vi "Stability.vi"() -> (0 "Done!":bool)   [LabVIEW 2013]
doc: "Performs stability measurements according to ATLAS ITk Quality Control Specifications."
uses:
  InstrControl/Switching/Switching.lvclass
  InstrControl/SupplyControl/SupplyControl.lvclass
  InstrControl/MultimeterControl/MultimeterControl.lvclass
  general_VIs/globals/QC_MeasurementSetup.vi
  general_VIs/globals/QC_RunInformation.vi
  InstrControl/InstrumentSetup.vi
  InstrControl/ArduinoControl/ArduinoControl.lvclass
  InstrControl/InstrControl.lvclass
  <vilib>/Analysis/NI_AALBase.lvlib
panel:
  out "No. of sensors":i32
  out "Current":dbl[](array[numeric]) caption="Current [nA]"
  out "Tgraph":cluster{u32[], dbl[]}[](graph)
  out "Igraph":cluster{u32[], dbl[]}[](graph)
  out "Tab Control 2":enum32{"Stability Setup", "Stability Scan"}(tab)
  in  "Use DUT switch?":bool=TRUE
  in  "Add Button":bool
  in  "New Button":bool
  out "DB Serial Nos.":string[](array[string])
  out "Channel Nos.":string[](array[string])
  in  "User:":string(combo)="Christoph"
  in  "Quit":bool
  in  "Continue":bool
  in  "enable T\ncorrection":bool
  in  "Base\nTemperature":dbl=20.0 format="%.1f"
  out "scan interval [s]":i32=10
  out "Test Duration":u32 format="%<%H:%M:%S>t"
  out "Voltage [V]":dbl format="%.1f"
  out "Temp.":dbl[](array[numeric]) caption="Temp. [°C]" format="%#.2f"
  out "RH":dbl[](array[numeric]) caption="RH [%]" format="%#.2f"
  in  "Scales":T1(ring)
  in  "Iscale":enum16{"nanoAmps", "microAmps", "milliAmps"}(ring)
  out "positive ramp?":bool
  out "Tab Control":enum32{"Stability Setup", "Stability Scan"}(tab)
  in  "Temperature":enum16{"Read Arduino", "Enter manually"}(ring)
  in  "Bias Supply":string(combo)="Keithley 2410"
  in  "Hardware Configurations":bool
  in  "DMM":string(combo)="Keithley 2000"
  in  "Set current limit?":bool
  in  "Current Limit [µA]":dbl=1000.0 min=0.0001 format="%.3f"
  in  "Test Duration IN":u32 caption="Test Duration" format="%<%H:%M:%S>t"
  in  "Measurement Configurations":bool
  in  "Voltage [V] IN":dbl caption="Voltage [V]"
  in  "scan interval [s] IN":i32=10 caption="scan interval [s]"
  in  "abort":bool
  out "Current Volts:":dbl format="%.2f"
  in  "quit (no save)":bool
  in  "Quit & Save":bool
  out "Bias On/Off:":bool
  out "STATUS 1":string
  out "Initiated:":string
  out "end of run":u32 format="%<%X\n%d/%m>T"
  out "runtime":u32 format="%<%H:%M:%S>t"
  out "Last reading at:":string
  # "University of\nCambridge"
  # "Strip Sensor QC: Current Stability"
  # "Vertical Scale:"
  # "DUT Description"
  # "Stability Scan parameters:"
  # "Temperature correction:"
  # "Measurement Configuration"
  # "Hardware"
  # "Current status:"
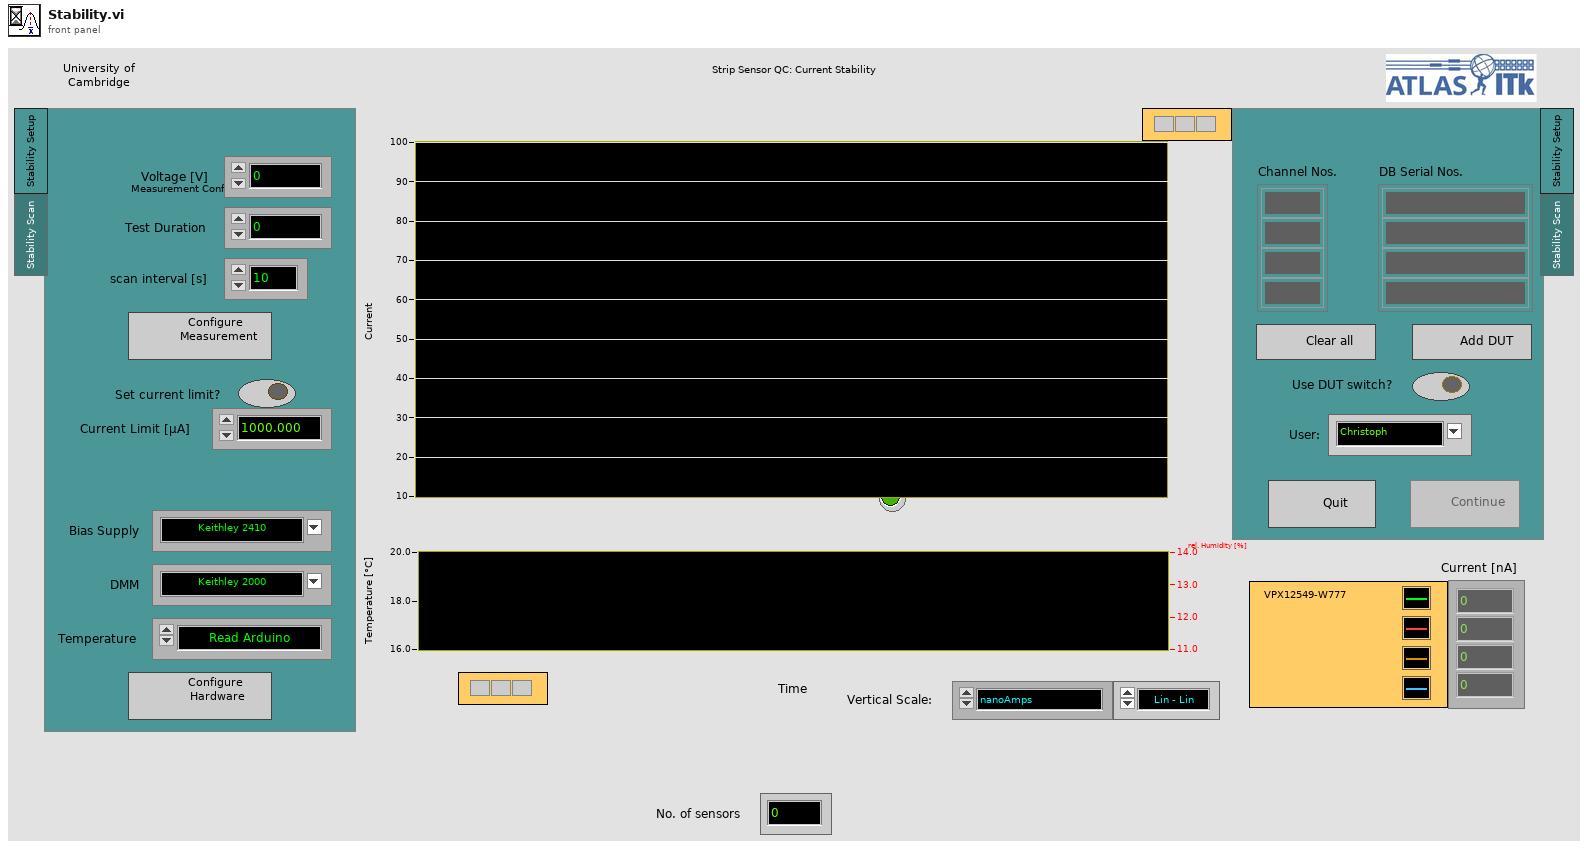
[diagram p1: front panel]
types:
  T1 = enum16{"Lin - Lin", "Log - Lin", "Lin - Log", "Log - log"}
  T2 = enum16{"Supply", "LCR", "Multimeter", "Switching"}
  T3 = enum32{"IV", "CV", "Stability", "Striptest", "Cis", "Ris", "PTP"}
  T4 = cluster{"Institute":string, "Manufacturers":string[], "Devices":string[], "Serialnumbers Lookup DB":string, "Data directory":string, "Backup & screenshot directory":string, "List of known users":string[], "Measurement switch not used":bool, "Measurement Switch":string, "DUT Switch":string, "Rseries IV [MOhm]":string, "Rshunt IV [MOhm]":string, "Rseries CV [MOhm]":string, "DC blocking Cap [µF]":string, "Rseries LCR [MOhm]":string, "Rseries stability [MOhm]":string, "Rshunt stability [MOhm]":string, "Rseries striptest bias [MOhm]":string, "Rseries strip pinhole [MOhm]":string}
  T5 = cluster{"Sensor Serial No.:":string, "Wafer:":string, "Batch:":string, "Manufacturer:":string, "Device Category:":string, "Database Serial No.:":string, "Date Initiated:":string, "Time Initiated:":string, "Test":string, "Probeplan used:":string, "End of Run comment:":string, "User:":string, "Vbias SMU":string, "LCR":string, "Test SMU":string, "Test DMM":string}
  T6 = cluster{"Supply":refnum<class "SupplyControl.lvclass">, "DMM":refnum<class "MultimeterControl.lvclass">, "DUT switch":refnum<class "Switching.lvclass">, "Arduino":refnum<class "ArduinoControl.lvclass">, "Measurement switch":refnum<class "Switching.lvclass">, "Voltage [V]":dbl, "Measurement Interval [s]":i32, "Test Duration":u32, "Ramp up steps [V]":dbl, "Ramp up Interval [s]":u32, "Ramp down steps [V]":dbl, "Ramp down Interval [s]":i32, "Set Current Limit?":bool, "Current Limit [µA]":dbl, "Temperature Readout":enum16{"Read Arduino", "Enter manually"}, "Supply Name":string, "DMM Name":string, "Maximum current fluctuation [%]":dbl, "Measurement switch used?":bool, "DUT switch used?":bool}
  T7 = enum16{"Reset", "Read Array", "Read Element", "Write Element", "Write Array", "Add Element", "Add Array"}
  T8 = cluster{"VISA address":refnum<visa-resource-name>, "T sensor":enum16{"SHT", "DS"}, "Arduino":refnum<class "ArduinoControl.lvclass">}
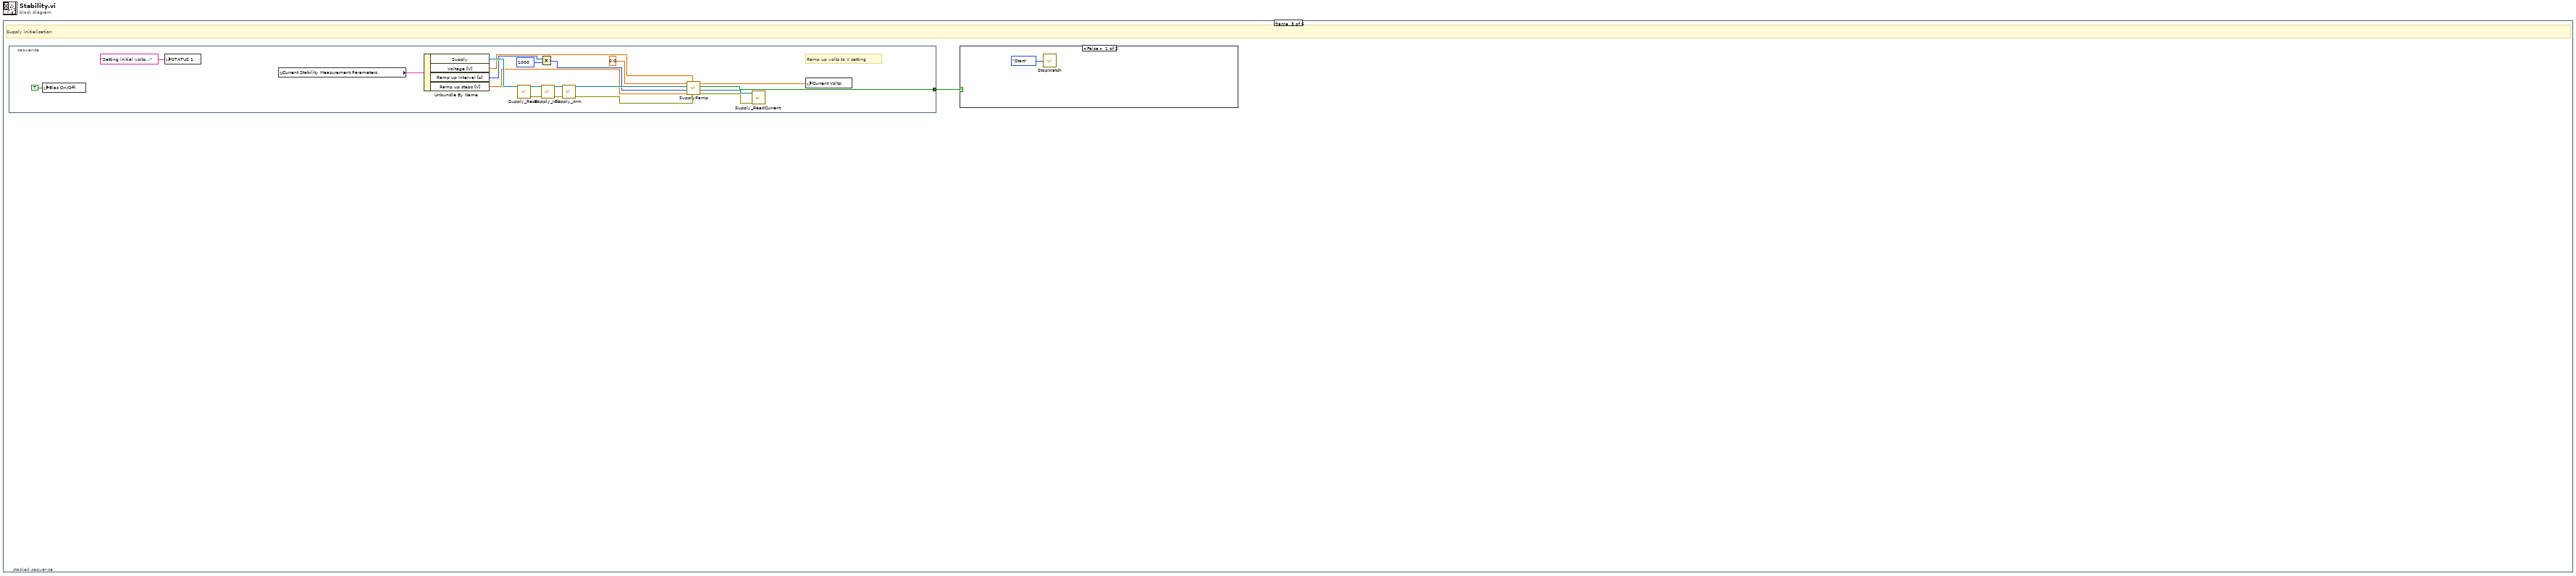
[diagram p0: block diagram]
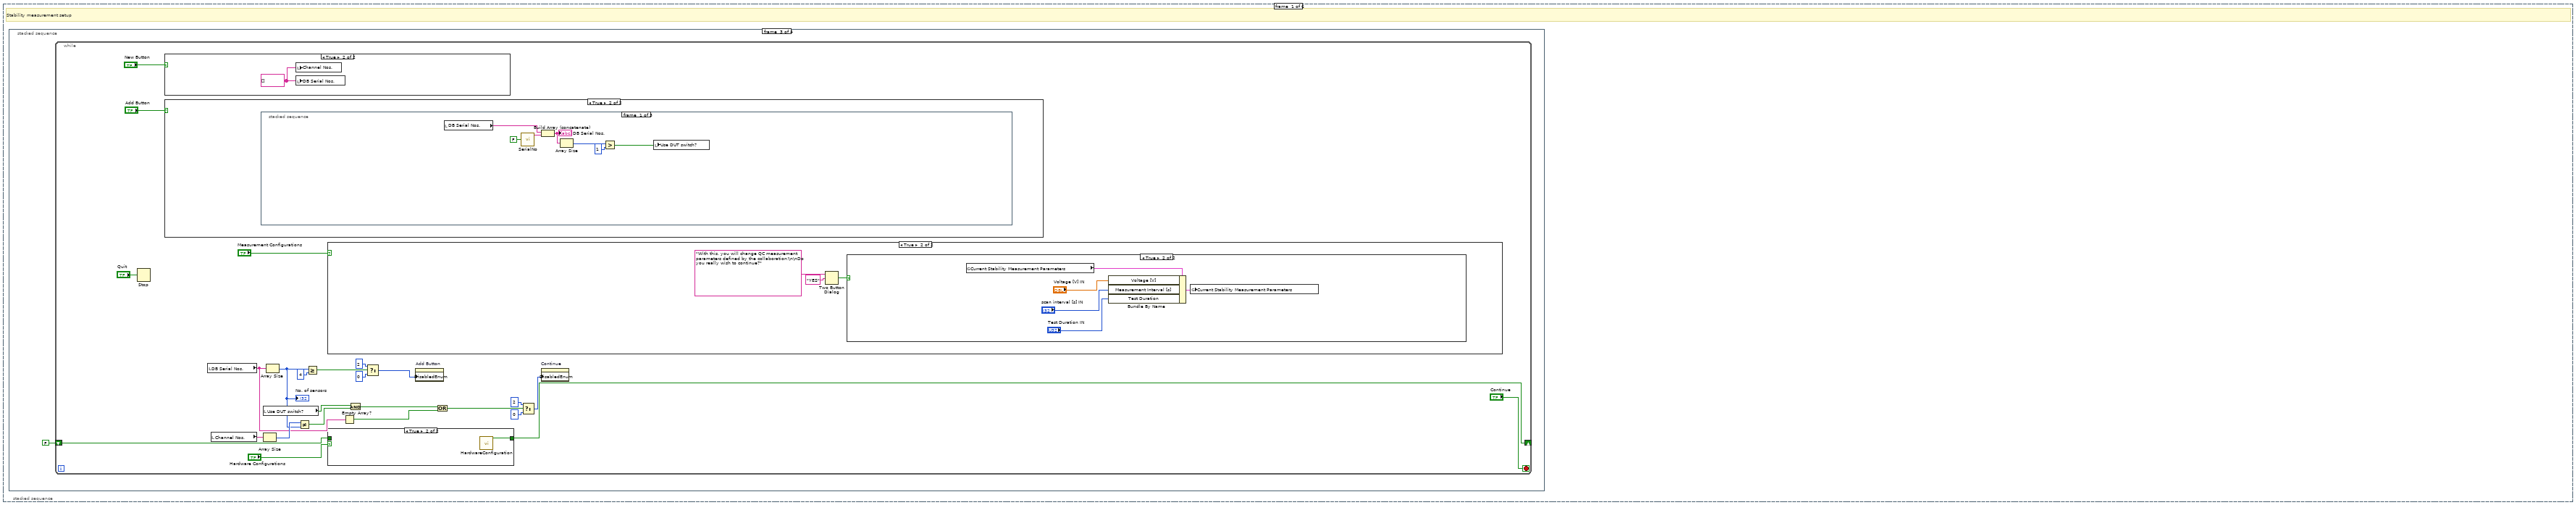
[diagram p2: hidden frame]
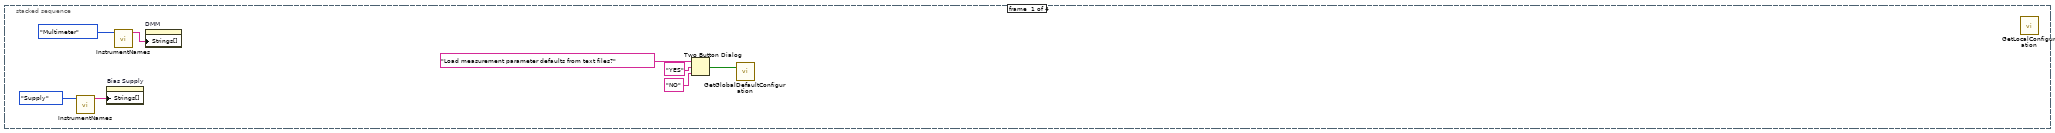
[diagram p3: hidden frame]
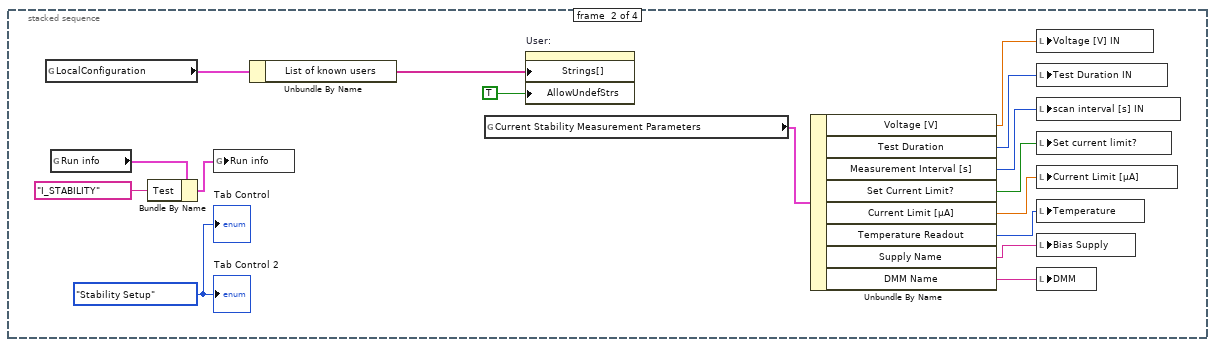
[diagram p4: hidden frame]
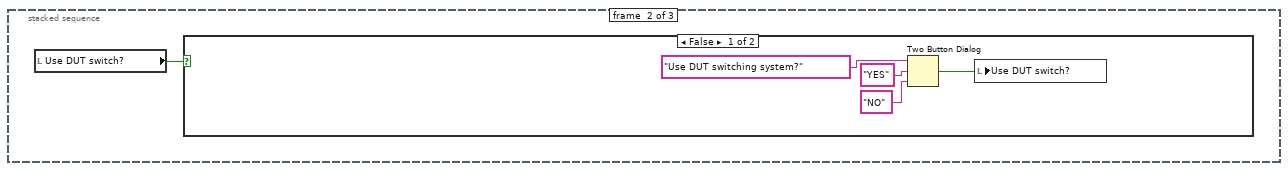
[diagram p7: hidden frame]
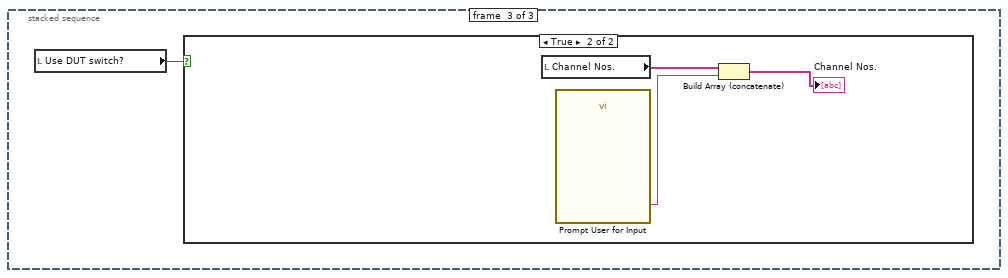
[diagram p9: hidden frame]
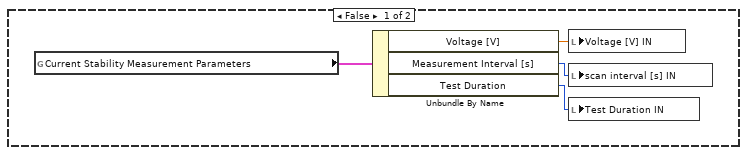
[diagram p12: hidden frame]
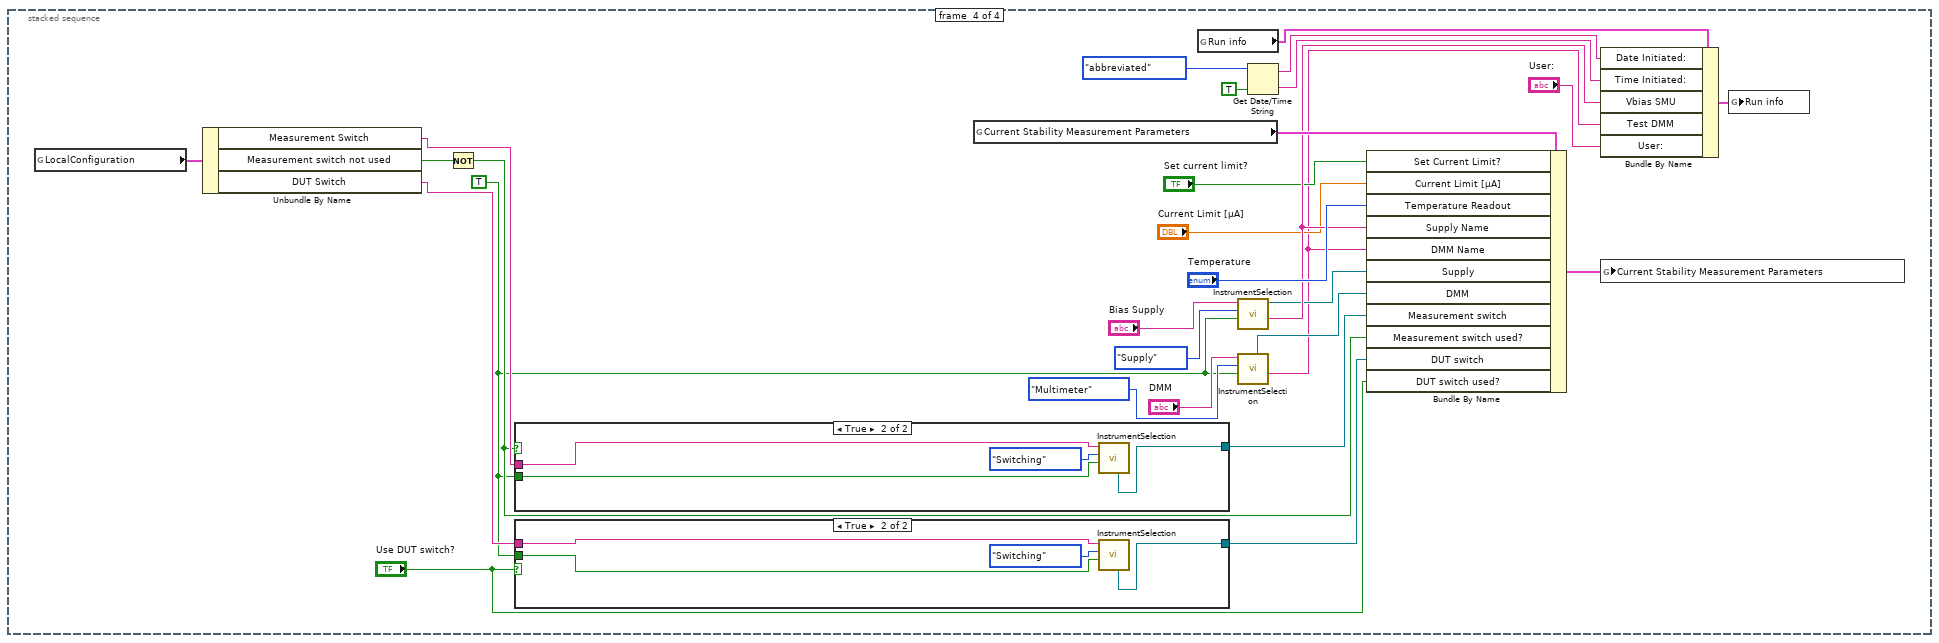
[diagram p14: hidden frame]
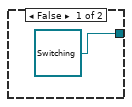
[diagram p15: hidden frame]
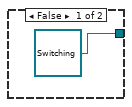
[diagram p16: hidden frame]
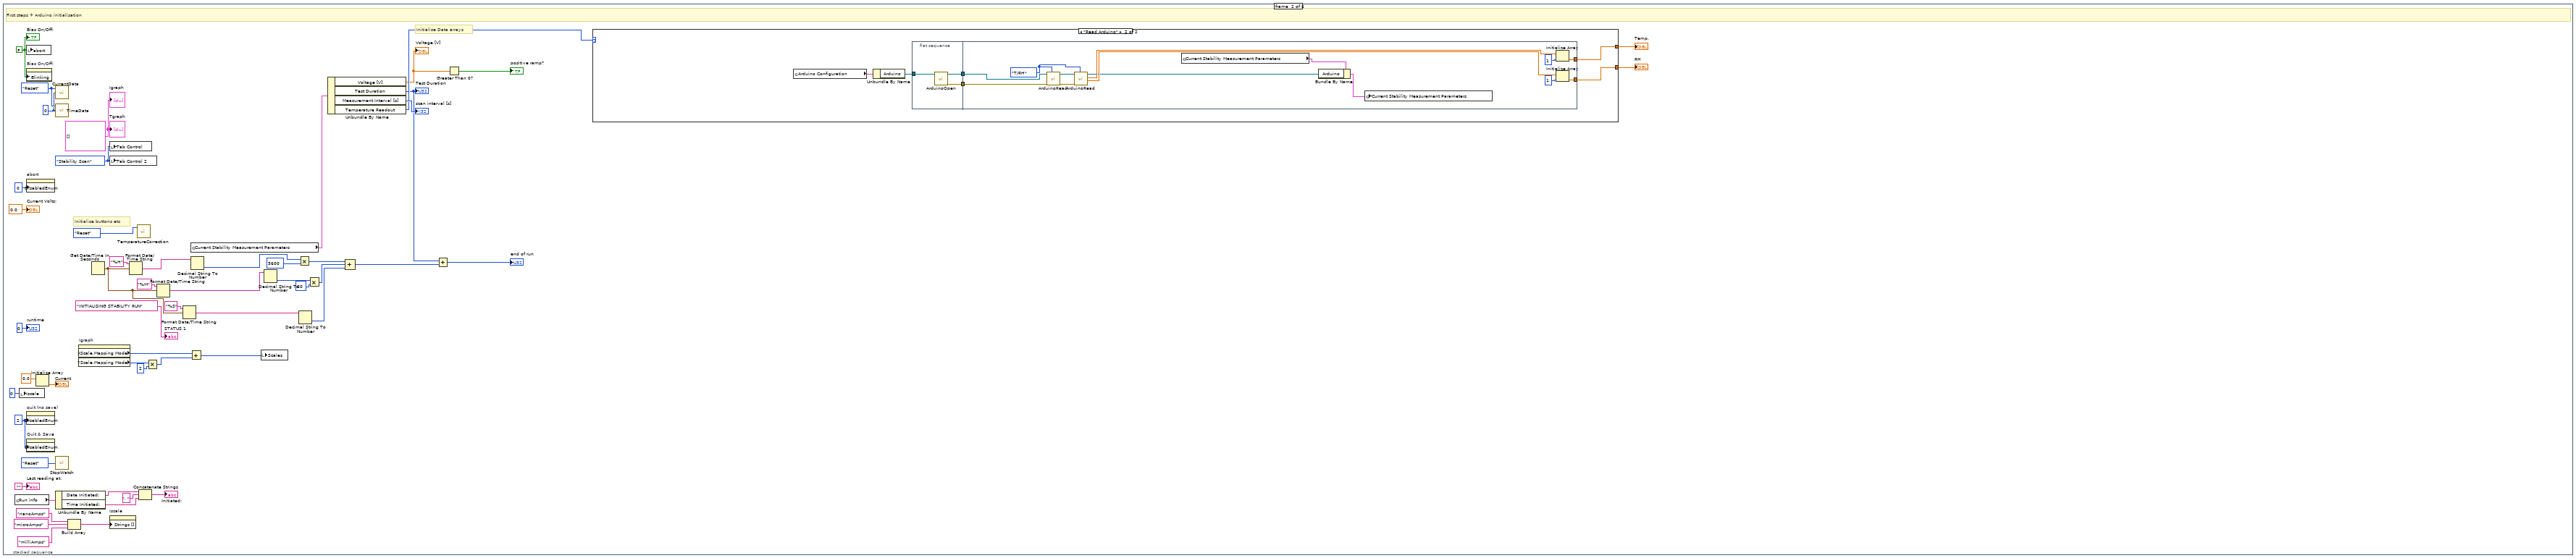
[diagram p17: hidden frame]
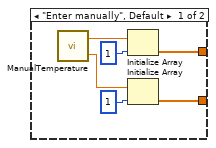
[diagram p18: hidden frame]
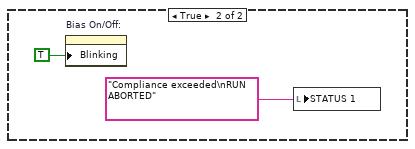
[diagram p19: hidden frame]
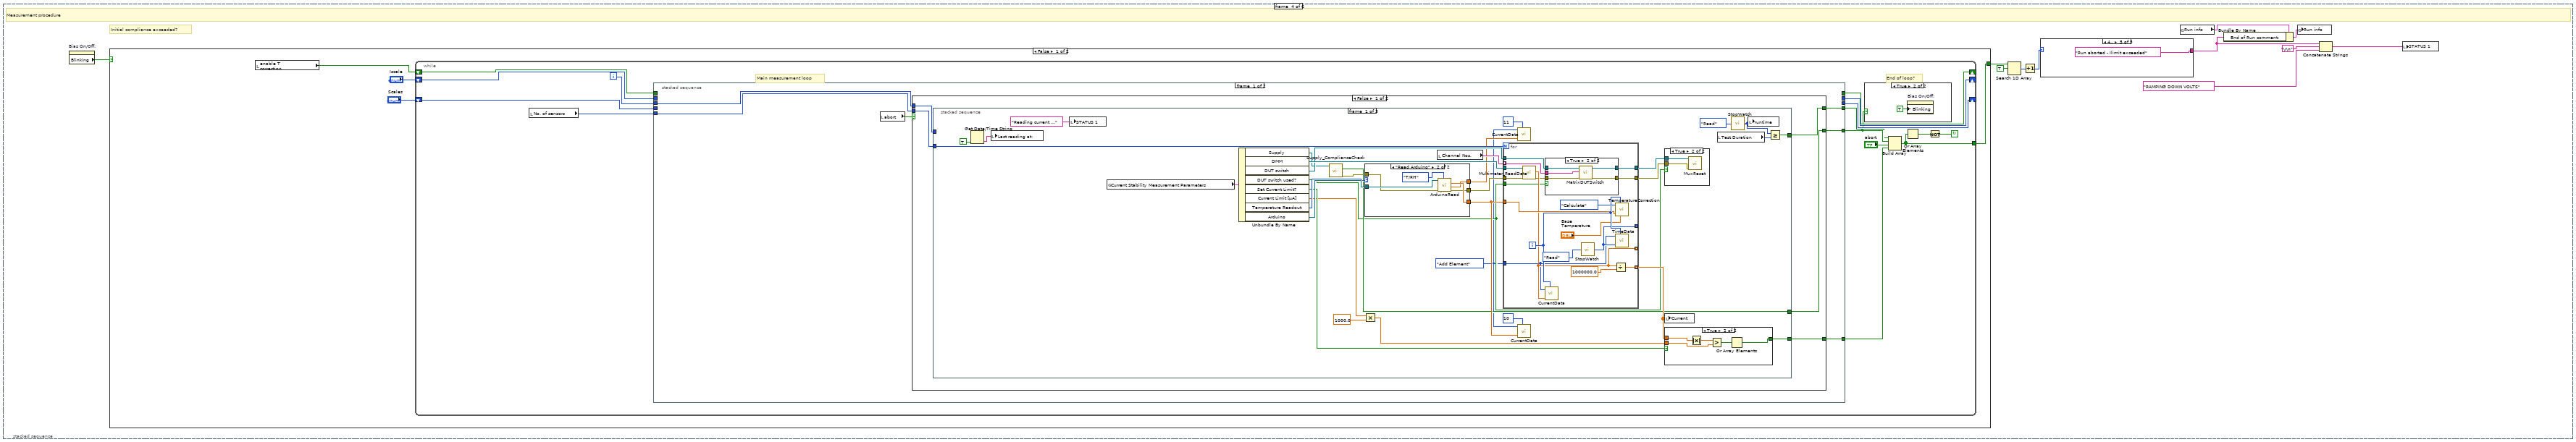
[diagram p20: hidden frame]
diagram:
  n1 = stacked-sequence {
    frame #0 {
      # "Stability measurement setup"
      n2 = stacked-sequence {
        frame #0 {
          n3 = call "InstrumentNames.vi"("Instrument type"=T2."Supply") -> ("Instrument names"=w7:string[])  [unwired: 9 in, 1 out]
          n4 = property on="Bias Supply" class="CmbBox"("Strings[]"=w7) -> ()  [unwired: 2 in, 2 out]
          n5 = call "InstrumentNames.vi"("Instrument type"=T2."Multimeter") -> ("Instrument names"=w2:string[])  [unwired: 9 in, 1 out]
          n6 = property on="DMM" class="CmbBox"("Strings[]"=w2) -> ()  [unwired: 2 in, 2 out]
          n7 = Two Button Dialog(message="Load measurement parameter defaults from text files?", 1:"NO", 2:"YES") -> (T button?=w6:bool)
          n8 = call "GetGlobalDefaultConfiguration.vi"("Read defaults?"=w6) -> ()  [unwired: 3 in]
          n9 = call "GetLocalConfiguration.vi"() -> ()  [unwired: 3 in, 1 out]
        }
        frame #1 {
          w13 = enum32{"Stability Setup", "Stability Scan"}."Stability Setup" ("Tab Control")
          n10 = global read "QC_RunInformation.vi" "LocalConfiguration"() -> (w10:T4)
          n11 = global read "QC_RunInformation.vi" "Run info"() -> (w19:T5)
          n12 = Bundle By Name(cluster=w19, "Test"="I_STABILITY") -> (w18:T5)
          n13 = global write "QC_RunInformation.vi" "Run info"(w18) -> ()
          n14 = Unbundle By Name(w10) -> ("List of known users"=w11:string[])
          n15 = global read "QC_MeasurementSetup.vi" "Current Stability Measurement Parameters"() -> (w22:T6)
          n16 = property on="User:" class="CmbBox"("Strings[]"=w11, "AllowUndefStrs"=TRUE) -> ()  [unwired: 2 in, 2 out]
          n17 = Unbundle By Name(w22) -> ("Voltage [V]"=w16:dbl, "Test Duration"=w15:u32, "Measurement Interval [s]"=w17:i32, "Set Current Limit?"=w21:bool, "Current Limit [µA]"=w20:dbl, "Temperature Readout"=w24:enum16{"Read Arduino", "Enter manually"}, "Supply Name"=w23:string, "DMM Name"=w9:string)
          n18 = local write "Voltage [V] IN"(w16) -> ()
          n19 = local write "Test Duration IN"(w15) -> ()
          n20 = local write "scan interval [s] IN"(w17) -> ()
          n21 = local write "Set current limit?"(w21) -> ()
          n22 = local write "Current Limit [µA]"(w20) -> ()
          n23 = local write "Temperature"(w24) -> ()
          n24 = local write "Bias Supply"(w23) -> ()
          n25 = local write "DMM"(w9) -> ()
          "Tab Control" <- w13
          "Tab Control 2" <- w13
        }
        frame #2 {
          n26 = while {
            shift-right: [w47] -> _
            shift-left: FALSE -> [w46]
            stop <- "Continue" stop-if-true
            n27 = Stop(stop? (T)="Quit") -> ()
            n28 = case shown="True" "New Button" {
              frame False {
              }
              frame True {
                w51 = string[] [] ("Channel Nos.")
                n29 = local write "Channel Nos."(w51) -> ()
                n30 = local write "DB Serial Nos."(w51) -> ()
              }
            }
            n31 = case shown="True" "Add Button" {
              frame False {
              }
              frame True {
                n32 = stacked-sequence {
                  frame #0 {
                    n33 = local read "DB Serial Nos."() -> (w57:string[])
                    n34 = call "SerialNo.vi"("Run uninterrupted?"=FALSE) -> ("DB serial number OUT"=w56:string)  [unwired: 7 in, 1 out]
                    n35 = Build Array (concatenate)(w57, w56) -> (w53:string[])
                    "DB Serial Nos." <- w53
                    n36 = Array Size(array=w53) -> (size(s)=w55:i32)
                    n37 = Greater?(x=w55, y=1) -> (0:w52:bool)
                    n38 = local write "Use DUT switch?"(w52) -> ()
                  }
                  frame #1 {
                    n39 = local read "Use DUT switch?"() -> (w59:bool)
                    n40 = case shown="False" w59 {
                      frame False {
                        n41 = Two Button Dialog(message="Use DUT switching system?", 1:"NO", 2:"YES") -> (T button?=w60:bool)
                        n42 = local write "Use DUT switch?"(w60) -> ()
                      }
                      frame True {
                      }
                    }
                  }
                  frame #2 {
                    n43 = local read "Use DUT switch?"() -> (w64:bool)
                    n44 = case shown="True" w64 {
                      frame False {
                      }
                      frame True {
                        n45 = local read "Channel Nos."() -> (w66:string[])
                        n46 = call "Prompt User for Input"() -> ("channel no."=w67:string)  [unwired: 17 in, 2 out]
                        n47 = Build Array (concatenate)(w66, w67) -> (→"Channel Nos.":string[])
                      }
                    }
                  }
                }
              }
            }
            n48 = local read "DB Serial Nos."() -> (w38:string[])
            n49 = local read "Channel Nos."() -> (w39:string[])
            n50 = local read "Use DUT switch?"() -> (w30:bool)
            n51 = Array Size(array=w39) -> (size(s)=w40:i32)
            n52 = Array Size(array=w38) -> (size(s)=w36:i32)
            "No. of sensors" <- w36
            n53 = Not Equal?(x=w40, y=w36) -> (x != y?=w31:bool)
            n54 = Greater Or Equal?(x=w36, y=4) -> (x >= y?=w32:bool)
            n55 = case shown="True" "Measurement Configurations" {
              frame False {
              }
              frame True {
                n56 = Two Button Dialog(message="With this, you will change QC measurement parameters defined by the collaboration!\n\nDo you really wish to continue?", 2:"YES") -> (T button?=w68:bool)  [unwired: 1 in]
                n57 = case shown="True" w68 {
                  frame False {
                    n58 = global read "QC_MeasurementSetup.vi" "Current Stability Measurement Parameters"() -> (w74:T6)
                    n59 = Unbundle By Name(w74) -> ("Voltage [V]"=w73:dbl, "Measurement Interval [s]"=w72:i32, "Test Duration"=w71:u32)
                    n60 = local write "Voltage [V] IN"(w73) -> ()
                    n61 = local write "scan interval [s] IN"(w72) -> ()
                    n62 = local write "Test Duration IN"(w71) -> ()
                  }
                  frame True {
                    n63 = global read "QC_MeasurementSetup.vi" "Current Stability Measurement Parameters"() -> (w79:T6)
                    n64 = Bundle By Name(cluster=w79, "Voltage [V]"="Voltage [V] IN", "Measurement Interval [s]"="scan interval [s] IN", "Test Duration"="Test Duration IN") -> (w78:T6)
                    n65 = global write "QC_MeasurementSetup.vi" "Current Stability Measurement Parameters"(w78) -> ()
                  }
                }
              }
            }
            n66 = case shown="True" "Hardware Configurations" {
              tunnel: [w80 w81] -> w47
              tunnel: w46 -> [w80 _]
              frame False {
              }
              frame True {
                n67 = call "HardwareConfiguration.vi"() -> ("configured?"=w81:bool)  [unwired: 11 in]
              }
            }
            n68 = Empty Array?(array=w38) -> (empty?=w29:bool)
            n69 = And(x=w30, y=w31) -> (x .and. y?=w28:bool)
            n70 = Select(t=2, s=w32, f=0) -> (s? t:f=w33:i32)
            n71 = property on="Add Button" class="Bool"("DisabledEnum"=w33) -> ()  [unwired: 2 in, 2 out]
            n72 = Or(x=w28, y=w29) -> (x .or. y?=w27:bool)
            n73 = Select(t=2, s=w27, f=0) -> (s? t:f=w43:i32)
            n74 = property on="Continue" class="Bool"("DisabledEnum"=w43) -> ()  [unwired: 2 in, 2 out]
          }
        }
        frame #3 {
          w82 = TRUE
          n75 = global read "QC_RunInformation.vi" "LocalConfiguration"() -> (w95:T4)
          n76 = Unbundle By Name(w95) -> ("Measurement Switch"=w93:string, "Measurement switch not used"=w94:bool, "DUT Switch"=w89:string)
          n77 = Not(x=w94) -> (.not. x?=w92:bool)
          n78 = case shown="True" w92 {
            tunnel: [refnum<class "Switching.lvclass"> refnum ("Switching") w119] -> w99
            tunnel: w82 -> [_ w118]
            tunnel: w93 -> [_ w117]
            frame False {
            }
            frame True {
              n79 = call "InstrumentSelection.vi"("Verify GPIB address"=w118, "Instrument type"=T2."Switching", "Instrument name IN"=w117) -> ("Switching"=w119:refnum<class "Switching.lvclass">)  [unwired: 3 in, 5 out]
            }
          }
          n80 = case shown="True" "Use DUT switch?" {
            tunnel: w89 -> [_ w114]
            tunnel: w82 -> [_ w113]
            tunnel: [refnum<class "Switching.lvclass"> refnum ("Switching") w112] -> w86
            frame False {
            }
            frame True {
              n81 = call "InstrumentSelection.vi"("Verify GPIB address"=w113, "Instrument type"=T2."Switching", "Instrument name IN"=w114) -> ("Switching"=w112:refnum<class "Switching.lvclass">)  [unwired: 3 in, 5 out]
            }
          }
          n82 = global read "QC_MeasurementSetup.vi" "Current Stability Measurement Parameters"() -> (w109:T6)
          n83 = global read "QC_RunInformation.vi" "Run info"() -> (w96:T5)
          n84 = call "InstrumentSelection.vi"("Verify GPIB address"=w82, "Instrument type"=T2."Supply", "Instrument name IN"="Bias Supply") -> ("Instrument name OUT"=w101:string, "Supply"=w100:refnum<class "SupplyControl.lvclass">)  [unwired: 3 in, 4 out]
          n85 = call "InstrumentSelection.vi"("Verify GPIB address"=w82, "Instrument type"=T2."Multimeter", "Instrument name IN"="DMM") -> ("Instrument name OUT"=w84:string, "Multimeter"=w87:refnum<class "MultimeterControl.lvclass">)  [unwired: 3 in, 4 out]
          n86 = Get Date/Time String(date format (0)=enum16{"short", "long", "abbreviated"}."abbreviated", want seconds? (F)=TRUE) -> (date string=w98:string, time string=w97:string)  [unwired: 1 in]
          n87 = Bundle By Name(cluster=w109, "Set Current Limit?"="Set current limit?", "Current Limit [µA]"="Current Limit [µA]", "Temperature Readout"="Temperature", "Supply Name"=w101, "DMM Name"=w84, "Supply"=w100, "DMM"=w87, "Measurement switch"=w99, "Measurement switch used?"=w92, "DUT switch"=w86, "DUT switch used?"="Use DUT switch?") -> (w110:T6)
          n88 = Bundle By Name(cluster=w96, "Date Initiated:"=w98, "Time Initiated:"=w97, "Vbias SMU"=w101, "Test DMM"=w84, "User:"="User:") -> (w106:T5)
          n89 = global write "QC_MeasurementSetup.vi" "Current Stability Measurement Parameters"(w110) -> ()
          n90 = global write "QC_RunInformation.vi" "Run info"(w106) -> ()
        }
      }
    }
    frame #1 {
      w121 = u32 0 ("Current reading No.")
      w149 = cluster{u32[], dbl[]}[] []
      w150 = enum32{"Stability Setup", "Stability Scan"}."Stability Scan" ("Tab Control")
      w122 = T7."Reset" ("Action")
      w160 = 2
      w159 = FALSE ("Visible")
      # "Initialise buttons etc"
      # "Initialise Data arrays"
      # "First steps + Arduino initialisation"
      n91 = global read "QC_RunInformation.vi" "Run info"() -> (w174:T5)
      n92 = local write "Iscale"(u16 0 ("Scale")) -> ()
      n93 = local write "abort"(w159) -> ()
      n94 = property on="Bias On/Off:" class="Bool (strict)"("Blinking"=w159) -> ()  [unwired: 2 in, 2 out]
      n95 = property on="abort" class="Bool (strict)"("DisabledEnum"=0) -> ()  [unwired: 2 in, 2 out]
      n96 = property on="quit (no save)" class="Bool"("DisabledEnum"=w160) -> ()  [unwired: 2 in, 2 out]
      n97 = property on="Quit & Save" class="Bool"("DisabledEnum"=w160) -> ()  [unwired: 2 in, 2 out]
      n98 = Initialize Array(0.0) -> (→"Current":dbl[])  [unwired: 1 in]
      n99 = call "CurrentData.vi"("Action"=w122, "Array Size / Index"=w121) -> ()  [unwired: 3 in, 2 out]
      n100 = call "TimeData.vi"("Action"=w122, "Array Size / Index"=w121) -> ()  [unwired: 3 in, 2 out]
      n101 = call "StopWatch.vi"("Action"=enum16{"Start", "Stop", "Read", "Reset"}."Reset") -> ()  [unwired: 5 out]
      n102 = Unbundle By Name(w174) -> ("Date Initiated:"=w128:string, "Time Initiated:"=w127:string)
      n103 = Build Array("nanoAmps", "microAmps", "milliAmps") -> (w171:string[])
      n104 = property on="Igraph" class="XYGraph (strict)"() -> ("XScale.Mapping Mode"=w148:u8, "YScale.Mapping Mode"=w147:u8)  [unwired: 2 in, 2 out]
      n105 = Get Date/Time In Seconds() -> (seconds since 1Jan1904=w144:timestamp)
      n106 = local write "Tab Control"(w150) -> ()
      n107 = local write "Tab Control 2"(w150) -> ()
      n108 = property on="Iscale" class="Enum (strict)"("Strings []"=w171) -> ()  [unwired: 2 in, 2 out]
      n109 = Format Date/Time String(time format string (%c)="%H", seconds (now)=w144) -> (date/time string=w142:string)  [unwired: 1 in]
      n110 = call "TemperatureCorrection.vi"("Action"=enum16{"Reset", "Calculate", "Correct"}."Reset") -> ()  [unwired: 4 in, 2 out]
      n111 = Concatenate Strings(w128, ", ", w127) -> (→"Initiated:":string)
      n112 = Multiply(x=w147, y=2) -> (x*y=w156:i32)
      n113 = Format Date/Time String(time format string (%c)="%M", seconds (now)=w144) -> (date/time string=w138:string)  [unwired: 1 in]
      n114 = Format Date/Time String(time format string (%c)="%S", seconds (now)=w144) -> (date/time string=w137:string)  [unwired: 1 in]
      n115 = Add(x=w148, y=w156) -> (x+y=w154:i32)
      n116 = global read "QC_MeasurementSetup.vi" "Current Stability Measurement Parameters"() -> (w152:T6)
      n117 = Decimal String To Number(string=w142) -> (number=w141:i32)  [unwired: 2 in, 1 out]
      n118 = local write "Scales"(w154) -> ()
      n119 = Decimal String To Number(string=w138) -> (number=w140:i32)  [unwired: 2 in, 1 out]
      n120 = Multiply(x=w141, y=3600) -> (x*y=w136:i32)
      n121 = Decimal String To Number(string=w137) -> (number=w134:i32)  [unwired: 2 in, 1 out]
      n122 = Multiply(x=w140, y=60) -> (x*y=w135:i32)
      n123 = Unbundle By Name(w152) -> ("Voltage [V]"=w158:dbl, "Test Duration"=w131:u32, "Measurement Interval [s]"=→"scan interval [s]":i32, "Temperature Readout"=w161:enum16{"Read Arduino", "Enter manually"})
      "Voltage [V]" <- w158
      "Test Duration" <- w131
      n124 = Compound Arithmetic op=ADD(w136, w135, w134) -> (w132:i32)
      n125 = Add(x=w131, y=w132) -> (x+y=→"end of run":u32)
      n126 = Greater Than 0?(x=w158) -> (x > 0?=→"positive ramp?":bool)
      n127 = case shown="\"Read Arduino\"" w161 {
        tunnel: [w180 w186] -> w163
        tunnel: [w179 w185] -> w153
        frame "Enter manually", Default {
          n128 = call "ManualTemperature.vi"() -> ("Humidity [%] out"=w175:dbl, "Temperature [°C] out"=w178:dbl)
          n129 = Initialize Array(w178, 1) -> (w180:dbl[])
          n130 = Initialize Array(w175, 1) -> (w179:dbl[])
        }
        frame "Read Arduino" {
          n131 = global read "InstrumentSetup.vi" "Arduino Configuration"() -> (w182:T8)
          n132 = Unbundle By Name(w182) -> ("Arduino"=w181:refnum<class "ArduinoControl.lvclass">)
          n133 = flat-sequence {
            tunnel: [w187] -> w184
            tunnel: [w189] -> w183
            tunnel: w181 -> [w188]
            tunnel: [w203] -> w186
            tunnel: [w200] -> w185
            tunnel: w184 -> [w194]
            tunnel: w183 -> [w193]
            frame #0 {
              n134 = call "ArduinoOpen.vi"("ArduinoControl in"=w188) -> ("error out"=w189:errorcluster, "ArduinoControl out"=w187:refnum<class "ArduinoControl.lvclass">)  [unwired: 9 in]
            }
            frame #1 {
              w190 = enum16{"T/RH", "Interlock", "Edgesense"}."T/RH" ("Arduino function")
              n135 = call "ArduinoRead.vi"("Arduino function"=w190, "error in (no error)"=w193, "ArduinoControl in"=w194) -> ("error out"=w192:errorcluster, "ArduinoControl out"=w191:refnum<class "ArduinoControl.lvclass">)  [unwired: 3 in, 4 out]
              n136 = call "ArduinoRead.vi"("Arduino function"=w190, "error in (no error)"=w192, "ArduinoControl in"=w191) -> ("rel. Humidity [%]"=w198:dbl, "Temperature [°C]"=w199:dbl, "ArduinoControl out"=w197:refnum<class "ArduinoControl.lvclass">)  [unwired: 3 in, 3 out]
              n137 = global read "QC_MeasurementSetup.vi" "Current Stability Measurement Parameters"() -> (w196:T6)
              n138 = Bundle By Name(cluster=w196, "Arduino"=w197) -> (w195:T6)
              n139 = global write "QC_MeasurementSetup.vi" "Current Stability Measurement Parameters"(w195) -> ()
              n140 = Initialize Array(w199, 1) -> (w203:dbl[])
              n141 = Initialize Array(w198, 1) -> (w200:dbl[])
            }
          }
        }
      }
      "Temp." <- w163
      "RH" <- w153
      "STATUS 1" <- "INITIALISING STABILITY RUN"
      "Bias On/Off:" <- w159
      "Last reading at:" <- ""
      "runtime" <- u32 0 ("Current reading No.")
      "Current Volts:" <- 0.0 ("Current Volts:")
      "Igraph" <- w149
      "Tgraph" <- w149
    }
    frame #2 {
      # "Supply initialisation"
      n142 = stacked-sequence {
        tunnel: [w210] -> w204
        frame #0 {
          # "Ramp up volts to V setting"
          n143 = local write "Bias On/Off:"(TRUE ("Compliance?")) -> ()
          n144 = local write "STATUS 1"("Setting initial volts..." ("STATUS 1")) -> ()
          n145 = global read "QC_MeasurementSetup.vi" "Current Stability Measurement Parameters"() -> (w220:T6)
          n146 = Unbundle By Name(w220) -> ("Supply"=w217:refnum<class "SupplyControl.lvclass">, "Voltage [V]"=w209:dbl, "Ramp up Interval [s]"=w206:u32, "Ramp up steps [V]"=w208:dbl)
          n147 = call-dynamic "Supply_Reset.vi"("SupplyControl in"=w217) -> ("error out"=w222:errorcluster, "SupplyControl out"=w224:refnum<class "SupplyControl.lvclass">)  [unwired: 9 in]
          n148 = Multiply(x=w206, y=1000) -> (x*y=w205:u32)
          n149 = call-dynamic "Supply_Init.vi"("error in (no error)"=w222, "SupplyControl in"=w224) -> ("error out"=w221:errorcluster, "SupplyControl out"=w223:refnum<class "SupplyControl.lvclass">)  [unwired: 8 in]
          n150 = call-dynamic "Supply_Arm.vi"("error in (no error)"=w221, "SupplyControl in"=w223) -> ("error out"=w213:errorcluster, "SupplyControl out"=w214:refnum<class "SupplyControl.lvclass">)  [unwired: 8 in]
          n151 = call "SupplyRamp.vi"("error in"=w213, "Requested Voltage"=w209, "Step Size"=w208, "Step Delay"=w205, "Supply IN"=w214, "Starting Voltage"=0.0) -> ("error out"=w211:errorcluster, "Supply OUT"=w212:refnum<class "SupplyControl.lvclass">, "Compliance exceeded"=w210:bool, "Current Voltage"=w216:dbl)  [unwired: 2 in]
          n152 = call-dynamic "Supply_ReadCurrent.vi"("error in (no error)"=w211, "SupplyControl in"=w212) -> ()  [unwired: 7 in, 3 out]
          n153 = local write "Current Volts:"(w216) -> ()
        }
      }
      n154 = case shown="False" w204 {
        frame False {
          n155 = call "StopWatch.vi"("Action"=enum16{"Start", "Stop", "Read", "Reset"}."Start") -> ()  [unwired: 5 out]
        }
        frame True {
          n156 = property on="Bias On/Off:" class="Bool (strict)"("Blinking"=TRUE) -> ()  [unwired: 2 in, 2 out]
          n157 = local write "STATUS 1"("Compliance exceeded\nRUN ABORTED") -> ()
        }
      }
    }
    frame #3 {
      # "Initial compliance exceeded?"
      # "Measurement procedure"
      n158 = property on="Bias On/Off:" class="Bool (strict)"() -> ("Blinking"=w238:bool)  [unwired: 2 in, 2 out]
      n159 = case shown="False" w238 {
        tunnel: [w247 w478] -> w237
        frame False {
          n160 = local read "enable T\ncorrection"() -> (w244:bool)
          n161 = while {
            shift-left: "Iscale" -> [w256]
            shift-right: [w253] -> _
            shift-left: "Scales" -> [w255]
            shift-right: [w252] -> _
            tunnel: [w260] -> w247
            shift-right: [w254] -> _
            shift-left: w244 -> [w258]
            i -> [w249]
            stop <- w261 continue-if-true
            # "Main measurement loop"
            # "End of loop?"
            n162 = local read "No. of sensors"() -> (w257:i32)
            n163 = stacked-sequence {
              tunnel: w258 -> [_ w403]
              tunnel: w257 -> [w267 w402]
              tunnel: w256 -> [_ w401]
              tunnel: w255 -> [_ w400]
              tunnel: [_ w399] -> w254
              tunnel: [_ w398] -> w253
              tunnel: [_ w397] -> w252
              tunnel: [w266 _] -> w251
              tunnel: [w265 _] -> w250
              tunnel: w249 -> [w264 _]
              tunnel: [w263 _] -> w248
              frame #0 {
                n164 = local read "abort"() -> (w268:bool)
                n165 = case shown="False" w268 {
                  tunnel: w267 -> [w273 _]
                  tunnel: [w272 w395] -> w266
                  tunnel: [w271 w395] -> w265
                  tunnel: w264 -> [w270 _]
                  tunnel: [w269 w395] -> w263
                  frame False {
                    n166 = stacked-sequence {
                      tunnel: w273 -> [w294 w363 _]
                      tunnel: [w285 _ _] -> w272
                      tunnel: [w283 _ _] -> w271
                      tunnel: w270 -> [_ _ w392]
                      tunnel: [w282 _ _] -> w269
                      frame #0 {
                        w274 = T7."Add Element" ("Action")
                        n167 = Get Date/Time String(want seconds? (F)=TRUE) -> (time string=w300:string)  [unwired: 2 in, 1 out]
                        n168 = local write "Last reading at:"(w300) -> ()
                        n169 = local write "STATUS 1"("Reading current ..." ("status")) -> ()
                        n170 = global read "QC_MeasurementSetup.vi" "Current Stability Measurement Parameters"() -> (w305:T6)
                        n171 = Unbundle By Name(w305) -> ("Supply"=w284:refnum<class "SupplyControl.lvclass">, "DMM"=w293:refnum<class "MultimeterControl.lvclass">, "DUT switch"=w292:refnum<class "Switching.lvclass">, "DUT switch used?"=w278:bool, "Set Current Limit?"=w299:bool, "Current Limit [µA]"=w297:dbl, "Temperature Readout"=w303:enum16{"Read Arduino", "Enter manually"}, "Arduino"=w304:refnum<class "ArduinoControl.lvclass">)
                        n172 = call-dynamic "Supply_ComplianceCheck.vi"("SupplyControl in"=w284) -> ("error out"=w275:errorcluster, "Compliance exceeded?"=w283:bool)  [unwired: 7 in, 2 out]
                        n173 = Multiply(x=w297, y=1000.0) -> (x*y=w296:dbl)
                        n174 = case shown="\"Read Arduino\"" w303 {
                          tunnel: [w343 w351] -> w286
                          tunnel: [w340 w350] -> w287
                          tunnel: w304 -> [_ w349]
                          tunnel: [w339 w347] -> w276
                          tunnel: w275 -> [w339 w346]
                          frame "Enter manually", Default {
                            n175 = local read "Temp."() -> (w345:dbl[])
                            n176 = local read "RH"() -> (w341:dbl[])
                            n177 = Index Array(array=w341, index=0) -> (element=w340:dbl)
                            n178 = Index Array(array=w345, index=0) -> (element=w343:dbl)
                          }
                          frame "Read Arduino" {
                            n179 = call "ArduinoRead.vi"("Arduino function"=enum16{"T/RH", "Interlock", "Edgesense"}."T/RH", "error in (no error)"=w346, "ArduinoControl in"=w349) -> ("error out"=w347:errorcluster, "rel. Humidity [%]"=w350:dbl, "Temperature [°C]"=w351:dbl)  [unwired: 3 in, 3 out]
                          }
                        }
                        n180 = local read "Channel Nos."() -> (w291:string[])
                        n181 = for {
                          N: w294 -> [_]
                          tunnel: w293 -> [w325]
                          tunnel: w292 -> [w316]
                          tunnel: w278 -> [w315]
                          tunnel: w291 -> [w317] mode=indexing
                          tunnel: [w319] -> _ mode=indexing
                          tunnel: [w318] -> _ mode=indexing
                          tunnel: [w314] -> w290 mode=indexing
                          tunnel: w286 -> [w321]
                          tunnel: [w320] -> w279
                          tunnel: [w310] -> w277
                          tunnel: w276 -> [w309]
                          tunnel: w274 -> [w308]
                          i -> [w323]
                          n182 = call-dynamic "Multimeter_ReadData.vi"("error in (no error)"=w309, "MultimeterControl in"=w325) -> ("error out"=w311:errorcluster, "Voltage in V"=w319:dbl)  [unwired: 7 in, 1 out]
                          n183 = case shown="True" w315 {
                            tunnel: w317 -> [_ w332]
                            tunnel: w316 -> [w327 w331]
                            tunnel: [w327 w330] -> w320
                            tunnel: w311 -> [w326 w329]
                            tunnel: [w326 w328] -> w310
                            frame False {
                            }
                            frame True {
                              n184 = call-dynamic "MatrixDUTSwitch.vi"("error in (no error)"=w329, "Channel #"=w332, "Switching in"=w331) -> ("error out"=w328:errorcluster, "Switching out"=w330:refnum<class "Switching.lvclass">)  [unwired: 7 in]
                            }
                          }
                          n185 = call "CurrentData.vi"("Action"=w308, "Array No."=w323, "Data IN"=w319) -> ()  [unwired: 2 in, 2 out]
                          n186 = call "StopWatch.vi"("Action"=enum16{"Start", "Stop", "Read", "Reset"}."Read") -> ("Time elapsed"=w318:u32)  [unwired: 4 out]
                          n187 = Divide(x=w319, y=1000000.0) -> (x/y=w314:dbl)
                          n188 = call "TemperatureCorrection.vi"("Action"=enum16{"Reset", "Calculate", "Correct"}."Calculate", "Sensor Index"=w323, "Actual temperature"=w321, "Correction temperature"="Base\nTemperature") -> ()  [unwired: 1 in, 2 out]
                          n189 = call "TimeData.vi"("Action"=w308, "Array No."=w323, "Data IN"=w318) -> ()  [unwired: 2 in, 2 out]
                        }
                        n190 = call "CurrentData.vi"("Action"=w274, "Array No."=u32 11, "Data IN"=w287) -> ()  [unwired: 2 in, 2 out]
                        n191 = call "CurrentData.vi"("Action"=w274, "Array No."=u32 10, "Data IN"=w286) -> ()  [unwired: 2 in, 2 out]
                        n192 = case shown="True" w278 {
                          tunnel: w279 -> [_ w307]
                          tunnel: w277 -> [_ w306]
                          frame False {
                          }
                          frame True {
                            n193 = call-dynamic "MuxReset.vi"("error in (no error)"=w306, "Switching in"=w307) -> ()  [unwired: 8 in, 2 out]
                          }
                        }
                        n194 = local write "Current"(w290) -> ()
                        n195 = case shown="True" w299 {
                          tunnel: w290 -> [_ w338]
                          tunnel: w296 -> [_ w336]
                          tunnel: [FALSE w334] -> w285
                          frame False {
                          }
                          frame True {
                            n196 = Absolute Value(x=w338) -> (abs(x)=w337:dbl[])
                            n197 = Greater?(x=w337, y=w336) -> (0:w335:bool[])
                            n198 = Or Array Elements(Boolean array=w335) -> (logical OR=w334:bool)
                          }
                        }
                        n199 = local read "Test Duration"() -> (w281:u32)
                        n200 = call "StopWatch.vi"("Action"=enum16{"Start", "Stop", "Read", "Reset"}."Read") -> ("Time elapsed"=w280:u32)  [unwired: 4 out]
                        n201 = local write "runtime"(w280) -> ()
                        n202 = Greater Or Equal?(x=w280, y=w281) -> (x >= y?=w282:bool)
                      }
                      frame #1 {
                        w361 = T7."Read Array" ("Action")
                        n203 = for {
                          N: w363 -> [_]
                          tunnel: [w371] -> w362 mode=indexing
                          i -> [w375]
                          w370 = T7."Read Array" ("Action")
                          n204 = Increment(x=w375) -> (x+1=w369:i32)
                          n205 = call "CurrentData.vi"("Action"=w370, "Array No."=w369) -> ("Array OUT"=w376:dbl[])  [unwired: 3 in, 1 out]
                          n206 = Absolute Value(x=w376) -> (abs(x)=w366:dbl[])
                          n207 = Divide(x=w366, y=1000000.0) -> (x/y=w364:dbl[])
                          n208 = case shown="True" "enable T\ncorrection" {
                            tunnel: w364 -> [w384 w388]
                            tunnel: [w384 w385] -> w374
                            tunnel: w369 -> [_ w386]
                            frame False {
                            }
                            frame True {
                              n209 = call "TemperatureCorrection.vi"("Action"=enum16{"Reset", "Calculate", "Correct"}."Correct", "Sensor Index"=w386, "Current IN"=w388) -> ("Current OUT"=w385:dbl[])  [unwired: 2 in, 1 out]
                            }
                          }
                          n210 = local read "Iscale"() -> (w367:enum16{"nanoAmps", "microAmps", "milliAmps"})
                          n211 = case shown="\"microAmps\"" w367 {
                            tunnel: [w377 w378 w382] -> w373
                            tunnel: w374 -> [w377 w380 w383]
                            frame .."nanoAmps" {
                            }
                            frame "microAmps" {
                              n212 = Divide(x=w380, y=1000.0) -> (x/y=w378:dbl[])
                            }
                            frame "milliAmps".. {
                              n213 = Divide(x=w383, y=1000000.0) -> (x/y=w382:dbl[])
                            }
                          }
                          n214 = call "TimeData.vi"("Action"=w370, "Array No."=w369) -> ("Array OUT"=w372:u32[])  [unwired: 3 in, 1 out]
                          n215 = Bundle("Array OUT"=w372, "Current OUT"=w373) -> (w371:cluster{"Array OUT":u32[], "Current OUT":dbl[]})  [unwired: 1 in]
                        }
                        n216 = call "CurrentData.vi"("Action"=w361, "Array No."=u32 10) -> ("Array OUT"=w356:dbl[])  [unwired: 3 in, 1 out]
                        n217 = call "CurrentData.vi"("Action"=w361, "Array No."=u32 11) -> ("Array OUT"=w355:dbl[])  [unwired: 3 in, 1 out]
                        n218 = call "TimeData.vi"("Action"=w361, "Array No."=0) -> ("Array OUT"=w357:u32[])  [unwired: 3 in, 1 out]
                        n219 = Bundle("Array OUT"=w357, "Array OUT"=w356) -> (w354:cluster{"Array OUT":u32[], "Array OUT":dbl[]})  [unwired: 1 in]
                        n220 = Bundle("Array OUT"=w357, "Array OUT"=w355) -> (w353:cluster{"Array OUT":u32[], "Array OUT":dbl[]})  [unwired: 1 in]
                        n221 = Build Array(w354, w353) -> (w352:cluster{"Array OUT":u32[], "Array OUT":dbl[]}[])
                        n222 = local write "Tgraph"(w352) -> ()
                        n223 = local write "Igraph"(w362) -> ()
                      }
                      frame #2 {
                        n224 = Quotient & Remainder(x=w392, y=10) -> (x-y*floor(x/y)=w390:i32)  [unwired: 1 out]
                        n225 = Equal To 0?(x=w390) -> (x = 0?=w389:bool)
                        n226 = case shown="True" w389 {
                          frame False {
                          }
                          frame True {
                            n227 = Current VI's Path() -> (path=w393:path)
                            n228 = call "SaveJPEG.vi"("Test"="Stability", "File Path Control"=w393) -> ()  [unwired: 1 in, 2 out]
                          }
                        }
                      }
                    }
                  }
                  frame True {
                    w395 = FALSE
                  }
                }
              }
              frame #1 {
                n229 = local read "scan interval [s]"() -> (w396:i32)
                n230 = Format Into String(format string="%d", w396) -> (resulting string=w408:string)  [unwired: 2 in, 1 out]
                n231 = Get Date/Time In Seconds() -> (seconds since 1Jan1904=w406:timestamp)
                n232 = To Double Precision Float(number=w406) -> (double precision float=w405:dbl)
                n233 = Concatenate Strings("Waiting for  ", w408, " seconds...") -> (w404:string)
                n234 = while {
                  tunnel: w405 -> [w419]
                  tunnel: w404 -> [w426]
                  tunnel: w402 -> [w438]
                  tunnel: w396 -> [w420]
                  shift-right: [w428] -> w397
                  shift-left: w400 -> [w431]
                  shift-right: [w429] -> w398
                  shift-left: w401 -> [w437]
                  shift-right: [w430] -> w399
                  shift-left: w403 -> [w436]
                  stop <- w415 continue-if-true
                  n235 = Get Date/Time In Seconds() -> (seconds since 1Jan1904=w423:timestamp)
                  n236 = Wait (ms)(milliseconds to wait=u32 100) -> ()  [unwired: 1 out]
                  n237 = local read "Scales"() -> (w428:T1)
                  n238 = To Double Precision Float(number=w423) -> (double precision float=w421:dbl)
                  n239 = local read "enable T\ncorrection"() -> (w430:bool)
                  n240 = Not Equal?(x=w431, y=w428) -> (x != y?=w432:bool)
                  n241 = Subtract(x=w421, y=w419) -> (x-y=w424:dbl)
                  n242 = local read "Iscale"() -> (w429:enum16{"nanoAmps", "microAmps", "milliAmps"})
                  n243 = local read "abort"() -> (w418:bool)
                  n244 = case shown="True" w432 {
                    tunnel: w428 -> [_ w441]
                    frame False {
                    }
                    frame True {
                      n245 = case shown="\"Log - log\".." w441 {
                        tunnel: [w442 1 0 w447] -> w440
                        tunnel: [w442 0 1 w447] -> w439
                        frame .."Lin - Lin" {
                          w442 = 0
                        }
                        frame "Log - Lin" {
                        }
                        frame "Lin - Log" {
                        }
                        frame "Log - log".. {
                          w447 = 1
                        }
                      }
                      n246 = property on="Igraph" class="XYGraph (strict)"("XScale.Mapping Mode"=w440) -> ()  [unwired: 2 in, 2 out]
                      n247 = property on="Igraph" class="XYGraph (strict)"("YScale.Mapping Mode"=w439, "YScale.Minimum"=w439) -> ()  [unwired: 2 in, 2 out]
                    }
                  }
                  n248 = Subtract(x=w420, y=w424) -> (x-y=w414:dbl)
                  n249 = Format Into String(format string="%d", w414) -> (resulting string=w413:string)  [unwired: 2 in, 1 out]
                  n250 = Not Equal?(x=w436, y=w430) -> (x != y?=w435:bool)
                  n251 = Not Equal?(x=w437, y=w429) -> (x != y?=w434:bool)
                  n252 = Not(x=w418) -> (.not. x?=w417:bool)
                  n253 = Greater Than 0?(x=w414) -> (x > 0?=w416:bool)
                  n254 = Or(x=w435, y=w434) -> (x .or. y?=w433:bool)
                  n255 = And(x=w417, y=w416) -> (x .and. y?=w415:bool)
                  n256 = case shown="True" w433 {
                    tunnel: w429 -> [_ w450]
                    tunnel: w438 -> [_ w448]
                    frame False {
                    }
                    frame True {
                      n257 = for {
                        N: w448 -> [_]
                        tunnel: w450 -> [w459]
                        tunnel: [w456] -> w449 mode=indexing
                        i -> [w462]
                        w455 = T7."Read Array" ("Action")
                        n258 = Increment(x=w462) -> (x+1=w454:i32)
                        n259 = call "CurrentData.vi"("Action"=w455, "Array No."=w454) -> ("Array OUT"=w463:dbl[])  [unwired: 3 in, 1 out]
                        n260 = local read "enable T\ncorrection"() -> (w461:bool)
                        n261 = Absolute Value(x=w463) -> (abs(x)=w453:dbl[])
                        n262 = Divide(x=w453, y=1000000.0) -> (x/y=w451:dbl[])
                        n263 = case shown="True" w461 {
                          tunnel: w451 -> [w471 w475]
                          tunnel: [w471 w472] -> w460
                          tunnel: w454 -> [_ w473]
                          frame False {
                          }
                          frame True {
                            n264 = call "TemperatureCorrection.vi"("Action"=enum16{"Reset", "Calculate", "Correct"}."Correct", "Sensor Index"=w473, "Current IN"=w475) -> ("Current OUT"=w472:dbl[])  [unwired: 2 in, 1 out]
                          }
                        }
                        n265 = case shown="\"microAmps\"" w459 {
                          tunnel: [w464 w465 w469] -> w458
                          tunnel: w460 -> [w464 w467 w470]
                          frame .."nanoAmps" {
                          }
                          frame "microAmps" {
                            n266 = Divide(x=w467, y=1000.0) -> (x/y=w465:dbl[])
                          }
                          frame "milliAmps".. {
                            n267 = Divide(x=w470, y=1000000.0) -> (x/y=w469:dbl[])
                          }
                        }
                        n268 = call "TimeData.vi"("Action"=w455, "Array No."=w454) -> ("Array OUT"=w457:u32[])  [unwired: 3 in, 1 out]
                        n269 = Bundle("Array OUT"=w457, "Current OUT"=w458) -> (w456:cluster{"Array OUT":u32[], "Current OUT":dbl[]})  [unwired: 1 in]
                      }
                      n270 = local write "Igraph"(w449) -> ()
                    }
                  }
                  n271 = Concatenate Strings(w426, "\r\n", "Timer status: ", w413) -> (w412:string)
                  n272 = local write "STATUS 1"(w412) -> ()
                }
              }
            }
            n273 = case shown="True" w250 {
              frame False {
              }
              frame True {
                n274 = property on="Bias On/Off:" class="Bool (strict)"("Blinking"=TRUE) -> ()  [unwired: 2 in, 2 out]
              }
            }
            n275 = Build Array(w248, w250, "abort", w251) -> (w260:bool[])
            n276 = Or Array Elements(Boolean array=w260) -> (logical OR=w262:bool)
            n277 = Not(x=w262) -> (.not. x?=w261:bool)
          }
        }
        frame True {
          w477 = FALSE
          # "compliance was exceeded when first voltage applied."
          # "Flag compliance as reason for end of run"
          n278 = local write "STATUS 1"("Run aborted - compliance exceeded.") -> ()
          n279 = Build Array(w477, TRUE, w477, w477) -> (w478:bool[])
        }
      }
      n280 = Search 1D Array(1D array=w237, element=TRUE) -> (index of element=w235:i32)  [unwired: 1 in]
      n281 = Increment(x=w235) -> (x+1=w234:i32)
      n282 = case shown="4.." w234 {
        tunnel: ["" "Run ended normally" "Compliance exceeded" "Run aborted - by user" "Run aborted - Ilimit exceeded"] -> w229
        frame ..0 {
        }
        frame 1 {
        }
        frame 2 {
          # "Determine reason for end of run."
        }
        frame 3 {
        }
        frame 4.. {
        }
      }
      n283 = global read "QC_RunInformation.vi" "Run info"() -> (w233:T5)
      n284 = Bundle By Name(cluster=w233, "End of Run comment:"=w229) -> (w228:T5)
      n285 = global write "QC_RunInformation.vi" "Run info"(w228) -> ()
      n286 = Concatenate Strings(w229, "\r\n", "RAMPING DOWN VOLTS") -> (w232:string)
      n287 = local write "STATUS 1"(w232) -> ()
    }
    frame #4 {
      # "Ramp down and switch off supply"
      n288 = stacked-sequence {
        frame #0 {
          # "Tie up loose ends. Set volts to zero and switch to standby"
          # "Ramp down volts now"
          n289 = global read "QC_MeasurementSetup.vi" "Current Stability Measurement Parameters"() -> (w489:T6)
          n290 = Unbundle By Name(w489) -> ("Supply"=w486:refnum<class "SupplyControl.lvclass">, "DUT switch"=w483:refnum<class "Switching.lvclass">, "Ramp down steps [V]"=w488:dbl, "Ramp down Interval [s]"=w487:i32, "DUT switch used?"=w482:bool)
          n291 = Multiply(x=w487, y=1000) -> (x*y=w491:i32)
          n292 = local read "Current Volts:"() -> (w494:dbl)
          n293 = call "SupplyRamp.vi"("Requested Voltage"=0.0, "Step Size"=w488, "Step Delay"=w491, "Supply IN"=w486, "Starting Voltage"=w494) -> ("error out"=w485:errorcluster, "Supply OUT"=w484:refnum<class "SupplyControl.lvclass">, "Current Voltage"=w492:dbl)  [unwired: 3 in, 1 out]
          n294 = local write "Current Volts:"(w492) -> ()
          n295 = call-dynamic "Supply_Stby.vi"("error in (no error)"=w485, "SupplyControl in"=w484) -> ("error out"=w481:errorcluster)  [unwired: 8 in, 1 out]
          n296 = case shown="True" w482 {
            tunnel: w483 -> [_ w496]
            tunnel: w481 -> [_ w495]
            frame False {
            }
            frame True {
              n297 = call-dynamic "MuxReset.vi"("error in (no error)"=w495, "Switching in"=w496) -> ()  [unwired: 8 in, 2 out]
            }
          }
        }
        frame #1 {
          w501 = 0
          n298 = local write "Bias On/Off:"(FALSE ("Visible")) -> ()
          n299 = local write "Current Volts:"(0.0 ("Current Volts:")) -> ()
          n300 = property on="Quit & Save" class="Bool"("DisabledEnum"=w501) -> ()  [unwired: 2 in, 2 out]
          n301 = property on="quit (no save)" class="Bool"("DisabledEnum"=w501) -> ()  [unwired: 2 in, 2 out]
          n302 = property on="abort" class="Bool (strict)"("DisabledEnum"=2) -> ()  [unwired: 2 in, 2 out]
          n303 = local write "STATUS 1"("Run finished. \nSave data?" ("STATUS 1")) -> ()
        }
        frame #2 {
          n304 = Current VI's Path() -> (path=w503:path)
          n305 = call "SaveJPEG.vi"("Test"="Stability", "File Path Control"=w503) -> ()  [unwired: 1 in, 2 out]
        }
      }
    }
    frame #5 {
      # "Loop and await decision on whether to save or junk data"
      # "Display and save data"
      n306 = local read "enable T\ncorrection"() -> (w504:bool)
      n307 = local read "Scales"() -> (w515:T1)
      n308 = local read "Iscale"() -> (w514:enum16{"nanoAmps", "microAmps", "milliAmps"})
      n309 = while {
        shift-left: w514 -> [w571]
        shift-right: [w570] -> _
        shift-left: w515 -> [w573]
        shift-right: [w572] -> _
        tunnel: ["Quit & Save"] -> w517
        tunnel: ["quit (no save)"] -> w516
        shift-right: [w561] -> _
        shift-left: w504 -> [w563]
        stop <- w568 continue-if-true
        n310 = local read "Scales"() -> (w572:T1)
        n311 = Not Equal?(x=w573, y=w572) -> (x != y?=w566:bool)
        n312 = case shown="True" w566 {
          tunnel: w572 -> [_ w604]
          frame False {
          }
          frame True {
            n313 = case shown="\"Log - log\".." w604 {
              tunnel: [w605 1 0 w610] -> w603
              tunnel: [w605 0 1 w610] -> w602
              frame .."Lin - Lin" {
                w605 = 0
              }
              frame "Log - Lin" {
              }
              frame "Lin - Log" {
              }
              frame "Log - log".. {
                w610 = 1
              }
            }
            n314 = property on="Igraph" class="XYGraph (strict)"("XScale.Mapping Mode"=w603) -> ()  [unwired: 2 in, 2 out]
            n315 = property on="Igraph" class="XYGraph (strict)"("YScale.Mapping Mode"=w602, "YScale.Minimum"=w602) -> ()  [unwired: 2 in, 2 out]
          }
        }
        n316 = local read "enable T\ncorrection"() -> (w561:bool)
        n317 = local read "Iscale"() -> (w570:enum16{"nanoAmps", "microAmps", "milliAmps"})
        n318 = Not Equal?(x=w563, y=w561) -> (x != y?=w564:bool)
        n319 = Not Equal?(x=w571, y=w570) -> (x != y?=w565:bool)
        n320 = Or(x=w564, y=w565) -> (x .or. y?=w562:bool)
        n321 = case shown="True" w562 {
          tunnel: w570 -> [_ w575]
          frame False {
          }
          frame True {
            n322 = local read "No. of sensors"() -> (w576:i32)
            n323 = for {
              N: w576 -> [_]
              tunnel: w575 -> [w585]
              tunnel: [w582] -> w574 mode=indexing
              i -> [w588]
              w581 = T7."Read Array" ("Action")
              n324 = Increment(x=w588) -> (x+1=w580:i32)
              n325 = call "CurrentData.vi"("Action"=w581, "Array No."=w580) -> ("Array OUT"=w589:dbl[])  [unwired: 3 in, 1 out]
              n326 = local read "enable T\ncorrection"() -> (w587:bool)
              n327 = Absolute Value(x=w589) -> (abs(x)=w578:dbl[])
              n328 = Divide(x=w578, y=1000000.0) -> (x/y=w577:dbl[])
              n329 = case shown="True" w587 {
                tunnel: w577 -> [w597 w601]
                tunnel: [w597 w598] -> w586
                tunnel: w580 -> [_ w599]
                frame False {
                }
                frame True {
                  n330 = call "TemperatureCorrection.vi"("Action"=enum16{"Reset", "Calculate", "Correct"}."Correct", "Sensor Index"=w599, "Current IN"=w601) -> ("Current OUT"=w598:dbl[])  [unwired: 2 in, 1 out]
                }
              }
              n331 = case shown="\"microAmps\"" w585 {
                tunnel: [w590 w591 w595] -> w584
                tunnel: w586 -> [w590 w593 w596]
                frame .."nanoAmps" {
                }
                frame "microAmps" {
                  n332 = Divide(x=w593, y=1000.0) -> (x/y=w591:dbl[])
                }
                frame "milliAmps".. {
                  n333 = Divide(x=w596, y=1000000.0) -> (x/y=w595:dbl[])
                }
              }
              n334 = call "TimeData.vi"("Action"=w581, "Array No."=w580) -> ("Array OUT"=w583:u32[])  [unwired: 3 in, 1 out]
              n335 = Bundle("Array OUT"=w583, "Current OUT"=w584) -> (w582:cluster{"Array OUT":u32[], "Current OUT":dbl[]})  [unwired: 1 in]
            }
            n336 = local write "Igraph"(w574) -> ()
          }
        }
        n337 = Not Or(1:"quit (no save)", 2:"Quit & Save") -> (0:w568:bool)
      }
      n338 = global read "QC_MeasurementSetup.vi" "Current Stability Measurement Parameters"() -> (w513:T6)
      n339 = Unbundle By Name(w513) -> ("Temperature Readout"=w512:enum16{"Read Arduino", "Enter manually"}, "Arduino"=w506:refnum<class "ArduinoControl.lvclass">)
      n340 = case shown="\"Read Arduino\"" w512 {
        tunnel: w506 -> [_ w560]
        frame "Enter manually", Default {
        }
        frame "Read Arduino" {
          n341 = call "ArduinoClose.vi"("ArduinoControl in"=w560) -> ()  [unwired: 9 in, 2 out]
        }
      }
      n342 = case shown="True" w516 {
        tunnel: [FALSE w612] -> w518
        frame False {
        }
        frame True {
          n343 = Two Button Dialog(message="Are you sure you don't want to save the data?", 1:"Quit" ("F button name (\"Cancel\")"), 2:"Save data" ("T button name (\"OK\")")) -> (T button?=w612:bool)
        }
      }
      n344 = Or(x=w517, y=w518) -> (x .or. y?=w511:bool)
      n345 = flat-sequence {
        tunnel: w511 -> [w521]
        tunnel: [w521] -> w507
        tunnel: [TRUE] -> w505
        frame #0 {
          n346 = local read "No. of sensors"() -> (w520:i32)
          n347 = local read "DB Serial Nos."() -> (w519:string[])
          n348 = for {
            N: w520 -> [_]
            tunnel: w521 -> [w524]
            tunnel: w519 -> [w526] mode=indexing
            i -> [w528]
            n349 = call "SerialNo.vi"("DB serial number IN"=w526, "Run uninterrupted?"=TRUE) -> ("Continue?"=w525:bool)  [unwired: 6 in, 1 out]
            n350 = And(x=w524, y=w525) -> (x .and. y?=w523:bool)
            n351 = case shown="True" w523 {
              tunnel: ["" w559] -> w537
              tunnel: [_ w549] -> w535
              tunnel: w528 -> [_ w541]
              frame False {
              }
              frame True {
                w545 = T7."Read Array" ("Action")
                n352 = local write "STATUS 1"("Saving Data ...") -> ()
                n353 = call "CurrentData.vi"("Action"=w545, "Array No."=u32 10 ("Action")) -> ("Array OUT"=w543:dbl[])  [unwired: 3 in, 1 out]
                n354 = call "CurrentData.vi"("Action"=w545, "Array No."=u32 11 ("Action")) -> ("Array OUT"=w542:dbl[])  [unwired: 3 in, 1 out]
                n355 = call "TimeData.vi"("Action"=w545, "Array No."=w541) -> ("Array OUT"=w544:u32[])  [unwired: 3 in, 1 out]
                n356 = call "CurrentData.vi"("Action"=w545, "Array No."=w541) -> ("Array OUT"=w540:dbl[])  [unwired: 3 in, 1 out]
                n357 = call <vilib>:"Std Deviation and Variance.vi"("X"=w543) -> ("mean"=w550:dbl)  [unwired: 1 in, 2 out]
                n358 = call <vilib>:"Std Deviation and Variance.vi"("X"=w542) -> ("mean"=w551:dbl)  [unwired: 1 in, 2 out]
                n359 = Build Array(w544, w543, w542, w540) -> (w554:dbl[][])
                n360 = Array Size(array=w540) -> (size(s)=w539:i32)
                n361 = Transpose 2D Array(2D array=w554) -> (transposed array=w553:dbl[][])
                n362 = call "SaveDataFile.vi"("Data Array"=w553, "Temperature"=w551, "Run uninterrupted?"=FALSE, "Humidity"=w550, "no. of arrays"=4, "Actual array lengths"=w539, "Array Titles"="Time[s] Temperature[C] Humidity[%] Shunt_voltage[mV]", "Strip Segment"="", "Arrays format"="%010.2f") -> ("Path + Filename OUT"=w559:string, "Error Out"=w549:errorcluster)  [unwired: 3 in, 2 out]
              }
            }
            n363 = global read "QC_MeasurementSetup.vi" "Current Stability Measurement Parameters"() -> (w536:T6)
            n364 = Unbundle By Name(w536) -> ("Maximum current fluctuation [%]"=w531:dbl)
            n365 = call "ScanFeedback.vi"("measurement type"=T3."Stability") -> ("Maximum current fluctuations"=w530:dbl)  [unwired: 4 in, 4 out]
            n366 = Greater Or Equal?(x=w530, y=w531) -> (x >= y?=w533:bool)
            n367 = call "WriteLogFile.vi"("Run uninterrupted?"=FALSE, "Automatic warning"="", "Data File"=w537, "Error In"=w535, "DUT passed?"=w533, "Value TechSpec criteria"=w530, "Files saved?"=w524) -> ()  [unwired: 4 in, 1 out]
          }
        }
      }
      n368 = Select(t="Run finished.\nData saved." ("STATUS 1"), s=w507, f="Run finished.\nData not saved." ("STATUS 1")) -> (s? t:f=w510:string)
      n369 = local write "STATUS 1"(w510) -> ()
      "Done!" <- w505
    }
  }
